vi "RANGE Update HHV.vi"(4 "HHV Propane":dbl, 5 "HHV Ref":refnum<vi>, 6 "HHV Natural Gas":dbl, 8 "error in (no error)":errorcluster, 9 "Manual HHV":bool, 11 "Display Bank":T1) -> (0 "error out":errorcluster)   [LabVIEW 2023]
uses:
  Type Definitions/RANGE Panel Data.ctl
  Drivers/Omega FMA-1600A Series Gas Flow Meter/Type Definitions/FMA1600A Gas Type.ctl
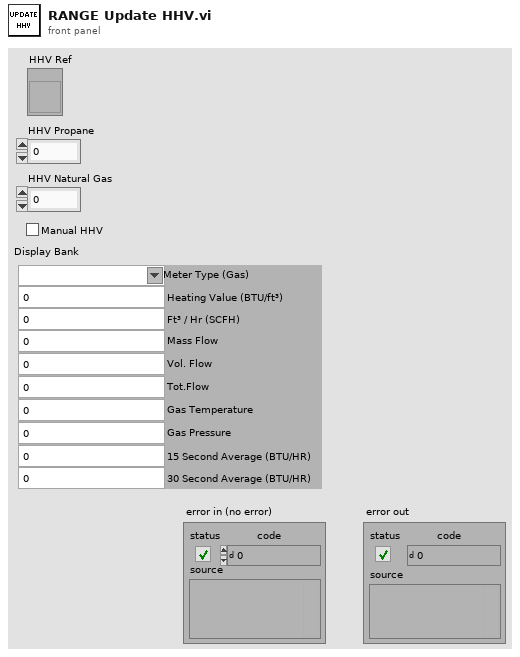
[diagram p1: front panel]
types:
  T1 = typedef "RANGE Panel Data.ctl" = cluster{"Meter Type (Gas)":T2, "Heating Value (BTU/ft³)":dbl, "Ft³ / Hr (SCFH)":dbl, "15 Second Average (BTU/HR)":dbl, "30 Second Average (BTU/HR)":dbl, "Mass Flow":dbl, "Vol. Flow":dbl, "Gas Temperature":dbl, "Gas Pressure":dbl, "Tot.Flow":dbl}
  T2 = typedef "FMA1600A Gas Type.ctl" = string
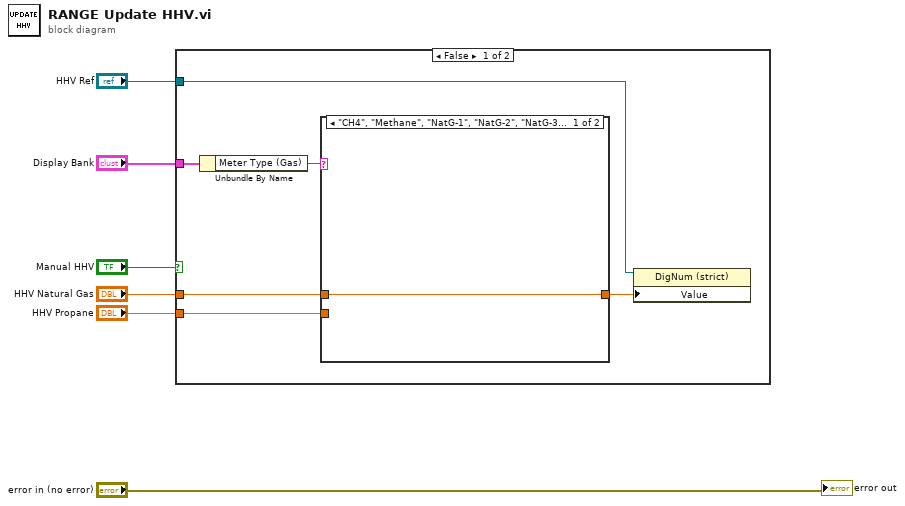
[diagram p0: block diagram]
diagram:
  n1 = case shown="False" "Manual HHV" {
    tunnel: "HHV Natural Gas" -> [w10 _]
    tunnel: "HHV Propane" -> [w9 _]
    tunnel: "Display Bank" -> [w8 _]
    tunnel: "HHV Ref" -> [w7 _]
    frame False {
      n2 = Unbundle By Name(w8) -> ("Meter Type (Gas)"=w12:T2)
      n3 = case shown="\"CH4\", \"Methane\", \"NatG-1\", \"NatG-2\", \"NatG-3\", Default" w12 {
        tunnel: w10 -> [w13 _]
        tunnel: w9 -> [_ w14]
        tunnel: [w13 w14] -> w11
        frame "CH4", "Methane", "NatG-1", "NatG-2", "NatG-3", Default {
        }
        frame "C3H8", "Propane" {
        }
      }
      n4 = property on="Property Node" class="DigNum (strict)"(reference=w7, "Value"=w11) -> ()  [unwired: 1 in, 2 out]
    }
    frame True {
    }
  }
  "error out" <- "error in (no error)"
